vi "windows_heater.vi"(0 "Power supply controls":refnum<vi>[][](array[refnum]), 1 "Window Heaters Physical Channels":T1, 2 "Switch Refnum":refnum<vi>, 3 "Stop! Refnum":refnum<vi>, 4 "Reset PS Error Refnum":refnum<vi>) -> ()   [LabVIEW 2017]
uses:
  <vilib>/Instr/_visa.llb/VISA Configure Serial Port (Instr).vi
  Input Channel Lists/window_heater_physical_channels.ctl
panel:
  out "error out":errorcluster
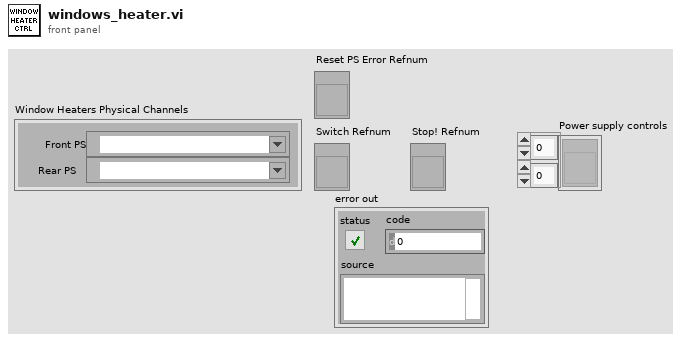
[diagram p1: front panel]
types:
  T1 = typedef "window_heater_physical_channels.ctl" = cluster{"Front PS":refnum<visa-resource-name>, "Rear PS":refnum<visa-resource-name>}
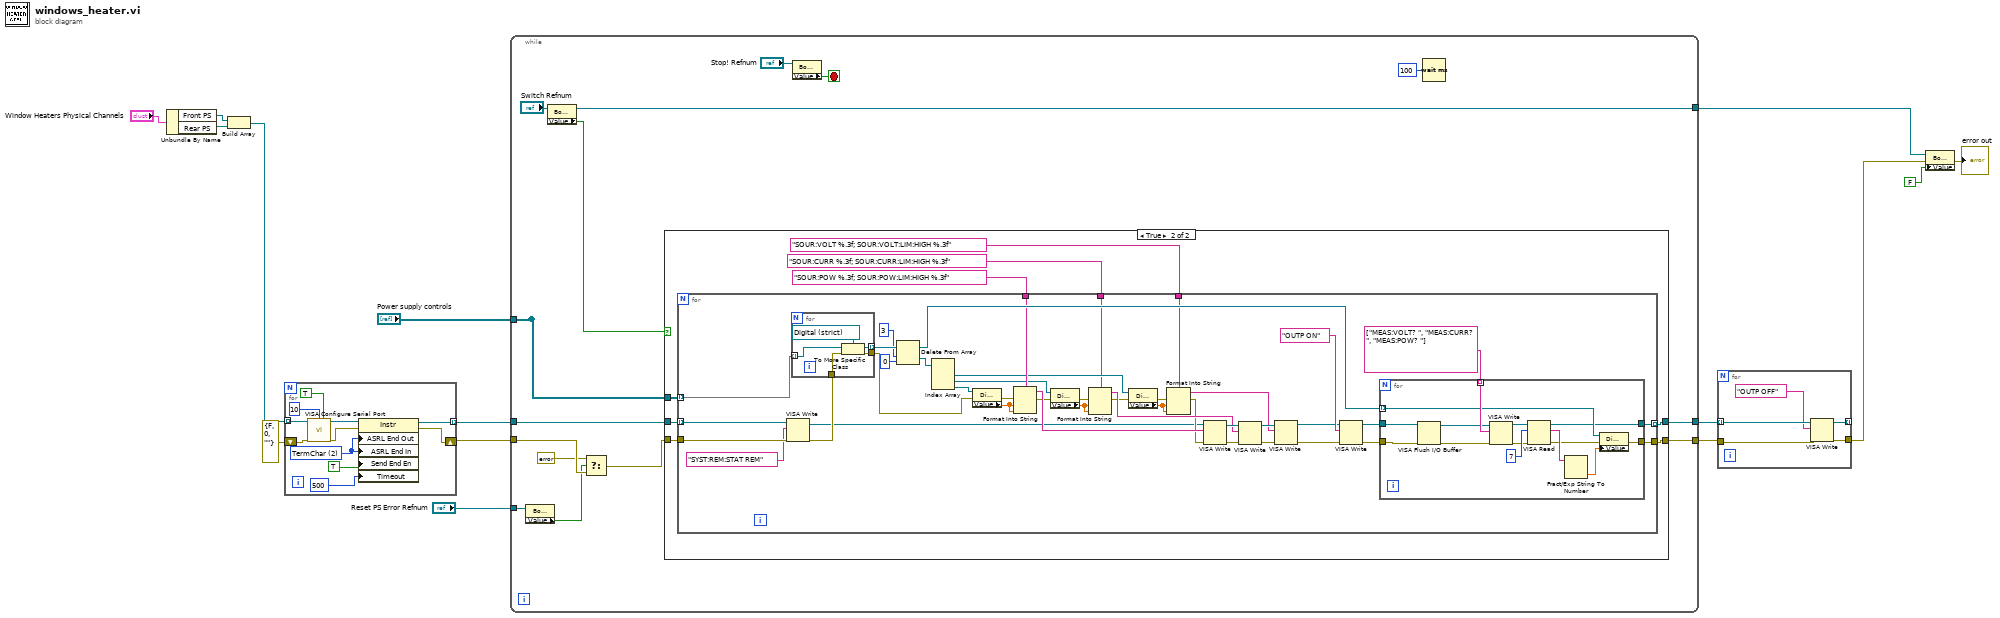
[diagram p0: block diagram]
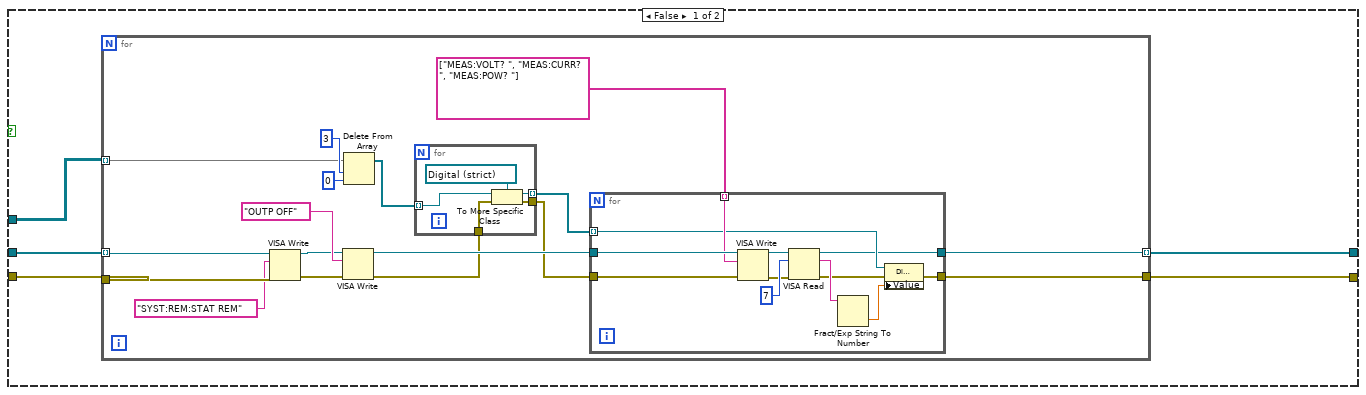
[diagram p2: hidden frame]
diagram:
  n1 = Unbundle By Name("Window Heaters Physical Channels") -> ("Front PS"=w12:refnum<visa-resource-name>, "Rear PS"=w11:refnum<visa-resource-name>)
  n2 = Build Array(w12, w11) -> (w10:refnum<visa-resource-name>[])
  n3 = for {
    tunnel: w10 -> [w26] mode=indexing
    tunnel: [w20] -> w9 mode=indexing
    shift-right: [w18] -> w7
    shift-left: errorcluster {"status"=FALSE, "code"=0, "source"=""} ("error out") -> [w19]
    w22 = u16 2 items=["None", "Last Bit", "TermChar", "Break"] ("Serial Settings:End Mode for Writes")
    n4 = call-poly "VISA Configure Serial Port"("VISA resource name"=w26, "termination char\n(0xA = '\\n' = LF)"=u8 10 ("termination char\n(0xA = '\\n' = LF)"), "Enable Termination\nChar (T)"=TRUE ("Enable Termination\nChar (T)"), "error in (no error)"=w19) -> ("VISA resource name out"=w24:refnum<visa-resource-name>, "error out"=w23:errorcluster)  [unwired: 10 in]
    n5 = property class="Instr"(reference=w24, error in=w23, "ASRL End Out"=w22, "ASRL End In"=w22, "Send End En"=TRUE ("Message Based Settings:Send End Enable"), "Timeout"=u32 500 ("General Settings:Timeout Value")) -> (reference out=w20:refnum<visa-resource-name>, error out=w18:errorcluster)
  }
  n6 = while {
    tunnel: [w39] -> w15
    tunnel: w9 -> [w37]
    tunnel: "Power supply controls" -> [w36]
    tunnel: w7 -> [w31]
    tunnel: [w36] -> _
    tunnel: [w34] -> w6
    tunnel: [w33] -> w5
    tunnel: "Reset PS Error Refnum" -> [w28]
    stop <- w41 stop-if-true
    n7 = property class="Bool (strict)"(reference=w28) -> ("Value"=w27:bool)  [unwired: 1 in, 2 out]
    n8 = property class="Bool (strict)"(reference="Switch Refnum") -> (reference out=w39:refnum<vi>, "Value"=w38:bool)  [unwired: 1 in, 1 out]
    n9 = Select(t=errorcluster {"status"=FALSE, "code"=0, "source"=""}, s=w27, f=w31) -> (s? t:f=w30:errorcluster)
    n10 = case shown="True" w38 {
      tunnel: w37 -> [w46 w88]
      tunnel: w36 -> [w42 w87]
      tunnel: w30 -> [w45 w86]
      tunnel: [w44 w85] -> w34
      tunnel: [w43 w84] -> w33
      frame False {
        n11 = for {
          tunnel: w46 -> [w48] mode=indexing
          tunnel: w45 -> [w49]
          tunnel: [w56] -> w44
          tunnel: [w57] -> w43 mode=indexing
          tunnel: w42 -> [w60] mode=indexing
          n12 = VISA Write(VISA resource name=w48, write buffer="SYST:REM:STAT REM", error in (no error)=w49) -> (VISA resource name out=w51:refnum<visa-resource-name>, error out=w50:errorcluster)  [unwired: 1 out]
          n13 = VISA Write(VISA resource name=w51, write buffer="OUTP OFF", error in (no error)=w50) -> (VISA resource name out=w59:refnum<visa-resource-name>, error out=w52:errorcluster)  [unwired: 1 out]
          n14 = Delete From Array(array=w60, length=3, index=0) -> (array with subset deleted=w55:refnum<vi>[])  [unwired: 1 out]
          n15 = for {
            tunnel: w55 -> [w67] mode=indexing
            tunnel: [w66] -> w54 mode=indexing
            tunnel: w52 -> [w65]
            tunnel: [w64] -> w53
            n16 = To More Specific Class(target class=refnum<vi> refnum ("Front Power Setpoint"), reference=w67, error in=w65) -> (specific class reference=w66:refnum<vi>, error out=w64:errorcluster)
          }
          n17 = for {
            tunnel: w54 -> [w73] mode=indexing
            tunnel: w59 -> [w80]
            tunnel: w53 -> [w79]
            tunnel: string[] ["MEAS:VOLT? ", "MEAS:CURR? ", "MEAS:POW? "] -> [w78] mode=indexing
            tunnel: [w70] -> w56
            tunnel: [w69] -> w57
            n18 = VISA Write(VISA resource name=w80, write buffer=w78, error in (no error)=w79) -> (VISA resource name out=w77:refnum<visa-resource-name>, error out=w75:errorcluster)  [unwired: 1 out]
            n19 = VISA Read(VISA resource name=w77, byte count=u32 7, error in (no error)=w75) -> (VISA resource name out=w69:refnum<visa-resource-name>, read buffer=w74:string, error out=w72:errorcluster)  [unwired: 1 out]
            n20 = Fract/Exp String To Number(string=w74) -> (number=w71:dbl)  [unwired: 3 in, 1 out]
            n21 = property class="DigNum (strict)"(reference=w73, error in=w72, "Value"=w71) -> (error out=w70:errorcluster)  [unwired: 1 out]
          }
        }
      }
      frame True {
        n22 = for {
          tunnel: w88 -> [w93] mode=indexing
          tunnel: w87 -> [w129] mode=indexing
          tunnel: w86 -> [w94]
          tunnel: [w122] -> w85
          tunnel: [w117] -> w84 mode=indexing
          tunnel: "SOUR:POW %.3f; SOUR:POW:LIM:HIGH %.3f" ("format string") -> [w114]
          tunnel: "SOUR:CURR %.3f; SOUR:CURR:LIM:HIGH %.3f" ("format string") -> [w98]
          tunnel: "SOUR:VOLT %.3f; SOUR:VOLT:LIM:HIGH %.3f" ("format string") -> [w97]
          n23 = VISA Write(VISA resource name=w93, write buffer="SYST:REM:STAT REM", error in (no error)=w94) -> (VISA resource name out=w90:refnum<visa-resource-name>, error out=w92:errorcluster)  [unwired: 1 out]
          n24 = for {
            tunnel: w129 -> [w148] mode=indexing
            tunnel: [w147] -> w127 mode=indexing
            tunnel: w92 -> [w146]
            tunnel: [w145] -> w128
            n25 = To More Specific Class(target class=refnum<vi> refnum ("Front Power Setpoint"), reference=w148, error in=w146) -> (specific class reference=w147:refnum<vi>, error out=w145:errorcluster)
          }
          n26 = Delete From Array(array=w127, length=3, index=0) -> (deleted portion=w115:refnum<vi>[], array with subset deleted=w126:refnum<vi>[])
          n27 = Index Array(array=w115) -> (element #1=w100:refnum<vi>, element #2=w110:refnum<vi>, element #3=w109:refnum<vi>)  [unwired: 3 in]
          n28 = property class="DigNum (strict)"(reference=w109, error in=w128) -> (error out=w121:errorcluster, "Value"=w113:dbl)  [unwired: 1 out]
          n29 = Format Into String(format string=w114, error in=w121, w113, w113) -> (resulting string=w120:string, error out=w104:errorcluster)  [unwired: 1 in]
          n30 = property class="DigNum (strict)"(reference=w110, error in=w104) -> (error out=w111:errorcluster, "Value"=w112:dbl)  [unwired: 1 out]
          n31 = Format Into String(format string=w98, error in=w111, w112, w112) -> (resulting string=w103:string, error out=w99:errorcluster)  [unwired: 1 in]
          n32 = property class="DigNum (strict)"(reference=w100, error in=w99) -> (error out=w102:errorcluster, "Value"=w101:dbl)  [unwired: 1 out]
          n33 = Format Into String(format string=w97, error in=w102, w101, w101) -> (resulting string=w96:string, error out=w91:errorcluster)  [unwired: 1 in]
          n34 = VISA Write(VISA resource name=w90, write buffer=w120, error in (no error)=w91) -> (VISA resource name out=w119:refnum<visa-resource-name>, error out=w118:errorcluster)  [unwired: 1 out]
          n35 = VISA Write(VISA resource name=w119, write buffer=w103, error in (no error)=w118) -> (VISA resource name out=w105:refnum<visa-resource-name>, error out=w106:errorcluster)  [unwired: 1 out]
          n36 = VISA Write(VISA resource name=w105, write buffer=w96, error in (no error)=w106) -> (VISA resource name out=w108:refnum<visa-resource-name>, error out=w107:errorcluster)  [unwired: 1 out]
          n37 = VISA Write(VISA resource name=w108, write buffer="OUTP ON", error in (no error)=w107) -> (VISA resource name out=w125:refnum<visa-resource-name>, error out=w124:errorcluster)  [unwired: 1 out]
          n38 = for {
            tunnel: w126 -> [w139] mode=indexing
            tunnel: w125 -> [w133]
            tunnel: w124 -> [w134]
            tunnel: string[] ["MEAS:VOLT? ", "MEAS:CURR? ", "MEAS:POW? "] -> [w144] mode=indexing
            tunnel: [w136] -> w122
            tunnel: [w135] -> w117
            n39 = VISA Flush I/O Buffer(VISA resource name=w133, error in (no error)=w134) -> (VISA resource name out=w132:refnum<visa-resource-name>, error out=w131:errorcluster)  [unwired: 1 in]
            n40 = VISA Write(VISA resource name=w132, write buffer=w144, error in (no error)=w131) -> (VISA resource name out=w143:refnum<visa-resource-name>, error out=w141:errorcluster)  [unwired: 1 out]
            n41 = VISA Read(VISA resource name=w143, byte count=u32 7, error in (no error)=w141) -> (VISA resource name out=w135:refnum<visa-resource-name>, read buffer=w140:string, error out=w138:errorcluster)  [unwired: 1 out]
            n42 = Fract/Exp String To Number(string=w140) -> (number=w137:dbl)  [unwired: 3 in, 1 out]
            n43 = property class="DigNum (strict)"(reference=w139, error in=w138, "Value"=w137) -> (error out=w136:errorcluster)  [unwired: 1 out]
          }
        }
      }
    }
    n44 = property class="Bool (strict)"(reference="Stop! Refnum") -> ("Value"=w41:bool)  [unwired: 1 in, 2 out]
    n45 = Wait (ms)(milliseconds to wait=u32 100) -> ()  [unwired: 1 out]
  }
  n46 = for {
    tunnel: w5 -> [w154] mode=indexing
    tunnel: w6 -> [w153]
    tunnel: [w152] -> w1
    tunnel: [w150] -> _ mode=indexing
    n47 = VISA Write(VISA resource name=w154, write buffer="OUTP OFF", error in (no error)=w153) -> (VISA resource name out=w150:refnum<visa-resource-name>, error out=w152:errorcluster)  [unwired: 1 out]
  }
  n48 = property class="Bool (strict)"(reference=w15, error in=w1, "Value"=FALSE) -> (error out=→"error out":errorcluster)  [unwired: 1 out]
